vi "get_data.vi"(4 "LabVIEW Web Service Request":refnum<class "Web Request.lvclass">) -> (2 "confidence":string, 3 "instrument":string)   [LabVIEW 2024]
uses:
  <vilib>/wsapi/Web Request.lvclass
panel:
  out "value":string
  out "standard output":string
  out "resulting string":string
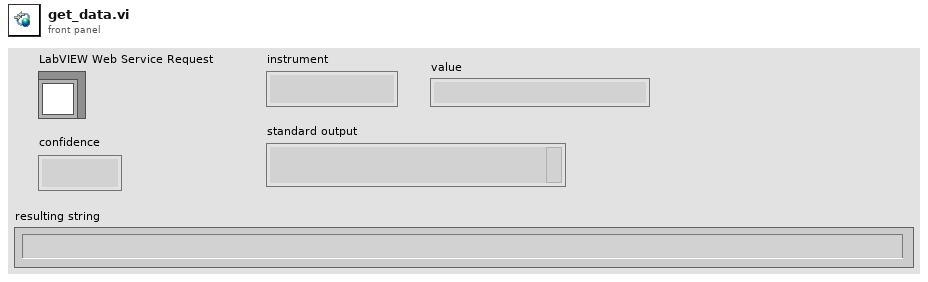
[diagram p1: front panel]
types:
  T1 = cluster{"instrument":string, "confidence":string}
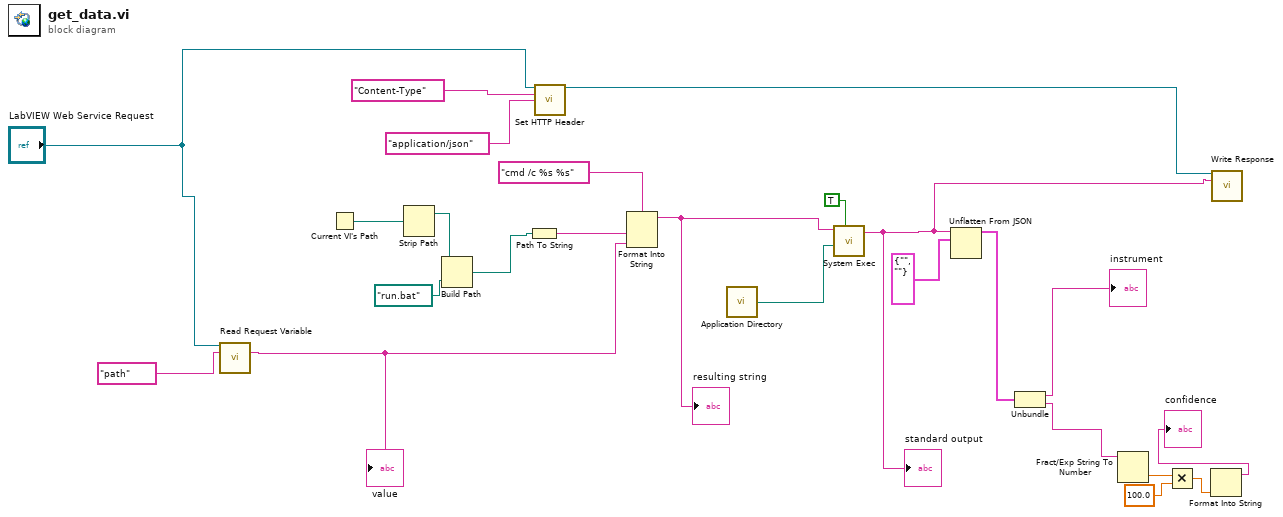
[diagram p0: block diagram]
diagram:
  n1 = call <vilib>:"Read Request Variable.vi"("LabVIEW Web Service Request"="LabVIEW Web Service Request", "variable name"="path") -> ("value"=w6:string)  [unwired: 11 in, 2 out]
  "value" <- w6
  n2 = Current VI's Path() -> (path=w16:path)
  n3 = Strip Path(path=w16) -> (stripped path=w15:path)  [unwired: 1 out]
  n4 = Build Path(base path=w15, name or relative path=path "run.bat") -> (appended path=w14:path)
  n5 = Path To String(path=w14) -> (string=w13:string)
  n6 = call <vilib>:"Set HTTP Header.vi"("LabVIEW Web Service Request"="LabVIEW Web Service Request", "header"="Content-Type", "header value"="application/json") -> ("LabVIEW Web Service Request out"=w3:refnum<class "Web Request.lvclass">)  [unwired: 11 in, 1 out]
  n7 = Format Into String "Format Into String"(format string="cmd /c %s %s", w13, w6) -> (resulting string=w23:string)  [unwired: 2 in, 1 out]
  "resulting string" <- w23
  n8 = call <vilib>:"Application Directory.vi"() -> ("Application Directory"=w17:path)
  n9 = call <vilib>:"System Exec.vi"("wait until completion? (T)"=TRUE, "working directory"=w17, "command line"=w23) -> ("standard output"=w5:string)  [unwired: 5 in, 3 out]
  "standard output" <- w5
  n10 = Unflatten From JSON(JSON string=w5, type and defaults=T1 {"instrument"="", "confidence"=""} ("Cluster")) -> (value=w21:T1)  [unwired: 5 in, 1 out]
  n11 = Unbundle(w21) -> ("instrument"=→"instrument":string, "confidence"=w18:string)
  n12 = Fract/Exp String To Number(string=w18) -> (number=w20:dbl)  [unwired: 3 in, 1 out]
  n13 = Multiply(x=w20, y=100.0) -> (x*y=w19:dbl)
  n14 = Format Into String(w19) -> (resulting string=→"confidence":string)  [unwired: 3 in, 1 out]
  n15 = call <vilib>:"Write Response.vi"("LabVIEW Web Service Request"=w3, "response string"=w5) -> ()  [unwired: 12 in, 2 out]
